vi "GetIntFeatureValue.vi"(9 "pFeatureName":string, 10 "handle":i64, 11 "error in (no error)":errorcluster) -> (2 "pIntValue":i64, 3 "error out":errorcluster)   [LabVIEW 2016]
uses:
  MVSDKmd.dll
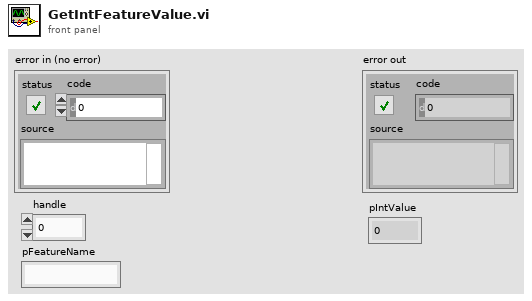
[diagram p1: front panel]
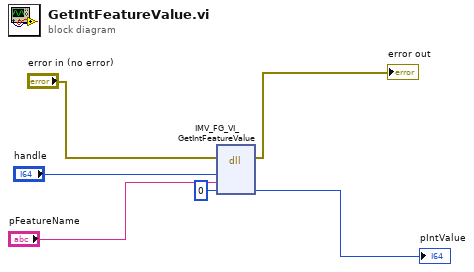
[diagram p0: block diagram]
diagram:
  n1 = dll-call lib="MVSDKmd.dll" fn="IMV_FG_VI_GetIntFeatureValue"(error in="error in (no error)", "handle"="handle", "pFeatureName"="pFeatureName", "pIntValue"=i64 0) -> (error out=→"error out":errorcluster, "pIntValue"=→"pIntValue":i64)  [unwired: 5 in, 1 out]
